vi "CSM DebugTool Dialog Ref(FGV).vi"(11 "VI Reference":refnum<vi>) -> (3 "VI Reference (Out)":refnum<vi>)   [LabVIEW 2017, in "CSM DebugTool Dialog.lvlib"]
uses:
  CSM DebugTool Dialog.lvlib
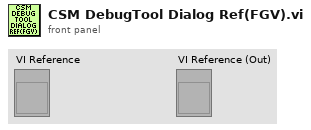
[diagram p1: front panel]
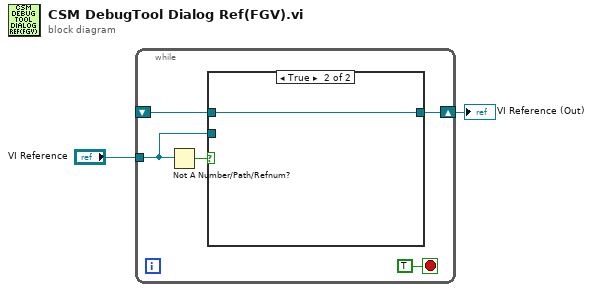
[diagram p0: block diagram]
diagram:
  n1 = while {
    shift-right: [w5] -> w1
    shift-left: _ -> [w4]
    tunnel: "VI Reference" -> [w3]
    stop <- TRUE stop-if-true
    n2 = Not A Number/Path/Refnum?(number/path/refnum=w3) -> (NaN/Path/Refnum?=w6:bool)
    n3 = case shown="True" w6 {
      tunnel: [w8 w9] -> w5
      tunnel: w4 -> [_ w9]
      tunnel: w3 -> [w8 _]
      frame False {
      }
      frame True {
      }
    }
  }
  "VI Reference (Out)" <- w1
